vi "Error Handler.vi"(7 "gRPC Server":refnum<class "gRPC Server.lvclass">, 8 "error_in":errorcluster) -> (0 "error out":errorcluster, 4 "Stop Loop":bool, 5 "gRPC Server out":refnum<class "gRPC Server.lvclass">)   [LabVIEW 2019, in "gRPC Server (template.proto).lvlib" / "gRPC Server.lvclass"]
uses:
  gRPC Server.lvclass
  <vilib>/addons/_Workers/Library/Classes/Worker/Worker.lvclass
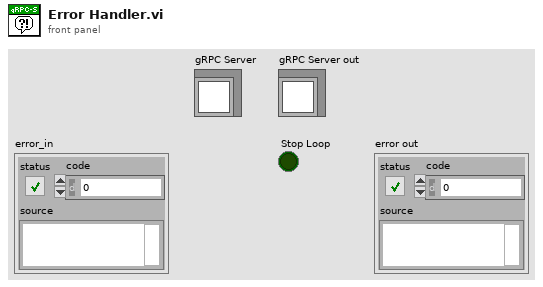
[diagram p1: front panel]
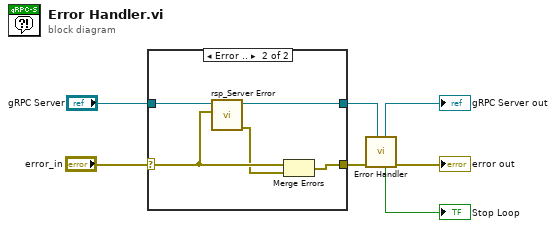
[diagram p0: block diagram]
diagram:
  n1 = case shown="Error .." "error_in" {
    selector: "error_in" -> [w8 w11]
    tunnel: "gRPC Server" -> [w9 w14]
    tunnel: [w9 w13] -> w3
    tunnel: [w8 w12] -> w2
    frame No Error {
    }
    frame Error {
      n2 = call "rsp_Server Error.vi"("Data in"=w11, "gRPC Server in"=w14) -> ("error out"=w10:errorcluster, "dup gRPC Server out"=w13:refnum<class "gRPC Server.lvclass">)  [unwired: 8 in]
      n3 = Merge Errors(w11, w10) -> (w12:errorcluster)
    }
  }
  n4 = call-parent "Error Handler.vi"("Worker"=w3, "error_in"=w2) -> ("error out"=→"error out":errorcluster, "Stop Loop"=→"Stop Loop":bool, "Worker out"=→"gRPC Server out":refnum<class "gRPC Server.lvclass">)  [unwired: 7 in]
